vi "misc-3.vi"() -> ()   [LabVIEW 2017]
panel:
  out "N° Iter":i32
  in  "Case?":enum16{"Polling", "Event"}(ring)
  in  "[ESC]":bool
  out "z":dbl(knob) caption="Sum" scale=0.0..20.0
  in  "y":dbl(slide) caption="Second number" scale=0.0..10.0
  in  "x":dbl(slide) caption="First number" scale=0.0..10.0
  # "Interaction with Front Panel: Polling technique vs Event structure"
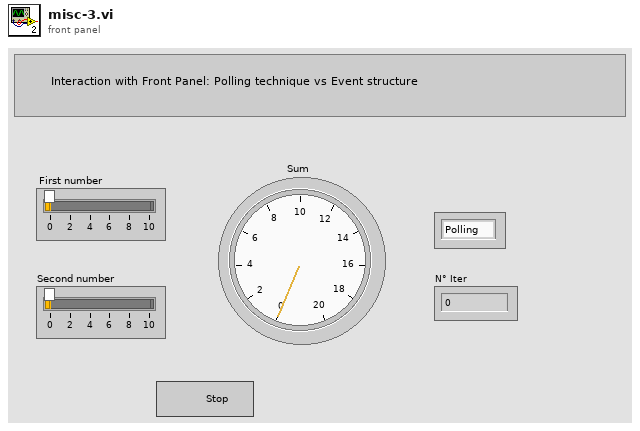
[diagram p1: front panel]
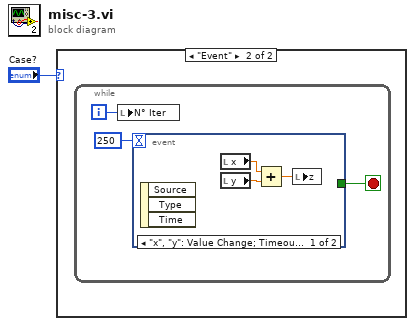
[diagram p0: block diagram]
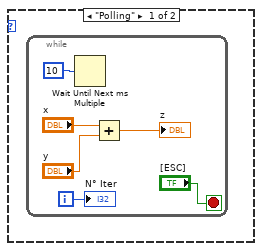
[diagram p2: hidden frame]
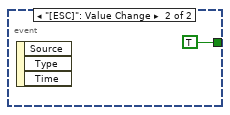
[diagram p3: hidden frame]
diagram:
  n1 = case shown="\"Event\"" "Case?" {
    frame "Polling" {
      n2 = while {
        i -> [w3]
        stop <- "[ESC]" stop-if-true
        n3 = Wait Until Next ms Multiple(millisecond multiple=u32 10 ("milliseconds to wait")) -> ()  [unwired: 1 out]
        n4 = Add(x="x", y="y") -> (x+y=→"z":dbl)
        "N° Iter" <- w3
      }
    }
    frame "Event" {
      n5 = while {
        i -> [w9]
        stop <- w10 stop-if-true
        n6 = local write "N° Iter"(w9) -> ()
        n7 = event shown="[0] \"x\", \"y\": Value Change;  Timeout" {
          selector: _ -> [_ _]
          dyn-events: _ -> [_ _]
          timeout: 250 -> [_ _]
          tunnel: [_ TRUE] -> w10
          event "x", "y": Value Change; Timeout {
            n8 = event-data() -> ()  [unwired: 1 in, 3 out]
            n9 = local read "x"() -> (w11:dbl)
            n10 = local read "y"() -> (w12:dbl)
            n11 = Add(x=w11, y=w12) -> (x+y=w13:dbl)
            n12 = local write "z"(w13) -> ()
          }
          event "[ESC]": Value Change {
            n13 = event-data() -> ()  [unwired: 1 in, 3 out]
          }
        }
      }
    }
  }
